vi "CC Install Simulation Config File.vi"() -> (2 "Hardware Config out":T1, 3 "new path":path)   [LabVIEW 2024]
uses:
  typedefs/CC cluster Hardware Config.ctl
  typedefs/CC cluster Device Index.ctl
panel:
  in  "OK Button":bool
  in  "Select Install Type":enum16{"Simulation", "Full Standard Hardware"}(ring)
  # "RIMAS Camera Control"
  # "No configuration file found. Select configuration from list below. Simulation mode will simulate all subsystem hardware. Full Standard Hardware attempts to communicate with all subsystems.\n\nHardware selections can be changed at anytime using the Settings-->Select Hardware menu option."
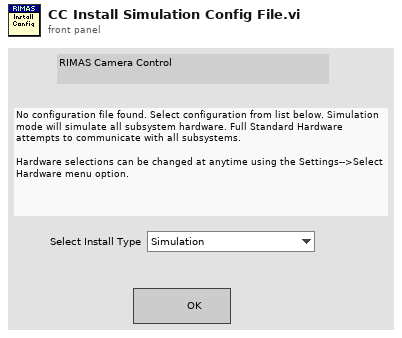
[diagram p1: front panel]
types:
  T1 = typedef "CC cluster Hardware Config.ctl" = cluster{"Installed Hardware":T2[]}
  T2 = typedef "CC cluster Device Index.ctl" = cluster{"Device Type Name":string, "Curr Device Name":string, "All Instances":string[]}
  T3 = enum32{"Invalid", "Standard", "Closed", "Hidden", "Minimized", "Maximized"}
diagram:
  w1 = "{\n  \"Arduino Focus Settings\":{\n    \"Homed\":[true,true],\n    \"Homing Parameters\":{\n      \"ACC/DECEL STEPS/SEC^2\":1000,\n      \"Direction\":false,\n      \"EN/DIS?\":true,\n      \"NUMBER OF  STEPS\":13000,\n      \"SPEED STEPS/SEC\":1000\n    },\n    \"Port\":\"ArduinoFocus\",\n    \"Positions\":[300,200]\n  },\n  \"Cryo Alarms\":{\n    \"Enabled\":false,\n    \"Reject Shutdown Temp\":40,\n    \"Reject Temp Warning\":20,\n    \"Temperature Error Max\":4\n  },\n  \"CryoCooler Settings\":{\n    \"Cryo Addr\":[\"Cooler1\",\"Cooler2\",\"Cooler3\"]\n  },\n  \"Detector Config PRIME\":{\"Detector\":0,\"Offsets\":[[0,0,0,0,0,0,0,0,0,0,0,0,0,0,0,0,0,0,0,0,0,0,0,0,0,0,0,0,0,0,0,0]],\"Detector Computer\":{\"Machine\":\"127.0.0.1\",\"Password\":\"R!MAS1grb\",\"FITS File Path\":\"/local/data/fermi-grb1/home/rimas/dev/h2rg/fitdat\",\"Port\":20750,\"Header Path\":\"/local/data/fermi-grb1/home/rimas/dev/h2rg/header\",\"Name\":\"PRIME\"},\"FITS hdr template0\":\"C:\\\\Users\\\\gsfcprime\\\\Documents\\\\LabVIEW Data\\\\FITS Templates\\\\header0.dat\",\"FITS hdr template1\":\"C:\\\\Users\\\\gsfcprime\\\\Documents\\\\LabVIEW Data\\\\FITS Templates\\\\header1.dat\",\"FITS Data File Path\":\"C:\\\\Users\\\\gsfcprime\\\\Documents\\\\LabVIEW Data\\\\PRIME FITS Images\",\"FITS Detector Settings\":{\"Exp Time Short\":1,\"# of Frames\":1,\"Exp Time Long\":2,\"# of Groups\":1,\"Object Name\":\"Auto\",\"Object\":\"\",\"Obs Type\":\"\",\"Image Type\":\"\",\"Observer\":\"\",\"Observer Affiliation\":\"\"},\"Sim Folder\":\"C:\\\\Users\\\\gsfcprime\\\\Documents\\\\LabVIEW Data\\\\PRIME Simulation FITS Images\",\"Integration Mode\":\"CDS\",\"Integration Time\":300,\"Frame Int Time\":3},\n  \"Detector Config RIMAS\":{\n    \"Detector Computer\":{\n      \"FITS File Path\":\"/local/data/fermi-grb1/home/rimas/dev/h2rg/fitdat\",\n      \"Header Path\":\"/local/data/fermi-grb1/home/rimas/dev/h2rg/header\",\n      \"Machine\":\"192.168.121.11\",\n      \"Name\":\"RIMAS\",\n      \"Password\":\"R!MAS1grb\",\n      \"Port\":44444\n    },\n    \"Detector\":0,\n    \"FITS Data File Path\":\"C:\\\\Users\\\\gsfcprime\\\\Documents\\\\LabVIEW Data\\\\PRIME FITS Images\",\n    \"FITS Detector Settings\":{\n      \"# of Frames\":1,\n      \"# of Groups\":1,\n      \"Exp Time Long\":2,\n      \"Exp Time Short\":1,\n      \"Image Type\":\"\",\n      \"Object Name\":\"\",\n      \"Object\":\"\",\n      \"Obs Type\":\"\",\n      \"Observer Affiliation\":\"\",\n      \"Observer\":\"\"\n    },\n    \"FITS hdr template0\":\"C:\\\\Users\\\\gsfcprime\\\\Documents\\\\LabVIEW Data\\\\FITS Templates\\\\header0.dat\",\n    \"FITS hdr template1\":\"C:\\\\Users\\\\gsfcprime\\\\Documents\\\\LabVIEW Data\\\\FITS Templates\\\\header1.dat\",\n    \"Frame Int Time\":0,\n    \"Integration Mode\":\"SSR\",\n    \"Integration Time\":0,\n    \"Offsets\":[\n      [\n        0,\n        0,\n        0,\n        0,\n        0,\n        0,\n        0,\n        0,\n        0,\n        0,\n        0,\n        0,\n        0,\n        0,\n        0,\n        0,\n        0,\n        0,\n        0,\n        0,\n        0,\n        0,\n        0,\n        0,\n        0,\n        0,\n        0,\n        0,\n        0,\n        0,\n        0,\n        0\n      ]\n    ],\n    \"Sim Folder\":\"C:\\\\Users\\\\gsfcprime\\\\Documents\\\\LabVIEW Data\\\\PRIME Simulation FITS Images\"\n  },\n  \"Detector Config Simulation\":{\n    \"Detector Computer\":{\n      \"FITS File Path\":\"/local/data/fermi-grb1/home/rimas/dev/h2rg/fitdat\",\n      \"Header Path\":\"/local/data/fermi-grb1/home/rimas/dev/h2rg/header\",\n      \"Machine\":\"\",\n      \"Name\":\"Simulation\",\n      \"Password\":\"R!MAS1grb\",\n      \"Port\":44444\n    },\n    \"Detector\":0,\n    \"FITS Data File Path\":\"C:\\\\Users\\\\gsfcprime\\\\Documents\\\\LabVIEW Data\\\\PRIME FITS Images\",\n    \"FITS Detector Settings\":{\n      \"# of Frames\":1,\n      \"# of Groups\":1,\n      \"Exp Time Long\":2,\n      \"Exp Time Short\":1,\n      \"Image Type\":\"\",\n      \"Object Name\":\"\",\n      \"Object\":\"\",\n      \"Obs Type\":\"\",\n      \"Observer Affiliation\":\"\",\n      \"Observer\":\"\"\n    },\n    \"FITS hdr template0\":\"C:\\\\Users\\\\gsfcprime\\\\Documents\\\\LabVIEW Data\\\\FITS Templates\\\\header0.dat\",\n    \"FITS hdr template1\":\"C:\\\\Users\\\\gsfcprime\\\\Documents\\\\LabVIEW Data\\\\FITS Templates\\\\header1.dat\",\n    \"Frame Int Time\":10,\n    \"Integration Mode\":\"SSR\",\n    \"Integration Time\":0,\n    \"Offsets\":[\n      [\n        0,\n        0,\n        0,\n        0,\n        0,\n        0,\n        0,\n        0,\n        0,\n        0,\n        0,\n        0,\n        0,\n        0,\n        0,\n        0,\n        0,\n        0,\n        0,\n        0,\n        0,\n        0,\n        0,\n        0,\n        0,\n        0,\n        0,\n        0,\n        0,\n        0,\n        0,\n        0\n      ]\n    ],\n    \"Sim Folder\":\"C:\\\\Users\\\\gsfcprime\\\\Documents\\\\LabVIEW Data\\\\PRIME Simulation FITS Images\"\n  },\n  \"Filter Wheel Settings RIMAS\":{\n    \"Addr\":\"ArduinoFilter\",\n    \"Default Speed\":200,\n    \"Filters\":[\n      {\n        \"Names\":[\"Grism\",\"Open\",\"Vph30\",\"Vph300\",\"Y\",\"J\"],\n        \"Relative Position\":[0,10000,17000,25000,33000,40000],\n        \"Size\":50000,\n        \"Wheel Name\":\"FW YJ\"\n      },\n      {\n        \"Names\":[\"Grism\",\"Open\",\"Vph30\",\"Vph300\",\"H\",\"K\"],\n        \"Relative Position\":[0,10000,17000,25000,33000,40000],\n        \"Size\":50000,\n        \"Wheel Name\":\"FW HK\"\n      },\n      {\n        \"Names\":[\n          \"K\",\n          \"Open\",\n          \"blank\",\n          \"Br-g\",\n          \"H2\",\n          \"2180\",\n          \"2190\"\n        ],\n        \"Relative Position\":[0,5560,11809,17908,23466,29016,34579],\n        \"Size\":40141,\n        \"Wheel Name\":\"Aux\"\n      },\n      {\n        \"Names\":[\n          \"blank\",\n          \"long\",\n          \"250 um\",\n          \"130 um\",\n          \"80 um\",\n          \"open\"\n        ],\n        \"Relative Position\":[0,5667,12889,20111,27333,34222],\n        \"Size\":40000,\n        \"Wheel Name\":\"Slit\"\n      }\n    ],\n    \"Homing\":[\n      {\n        \"Accel\":267,\n        \"Direction\":true,\n        \"Error Cnts\":300,\n        \"Homing Delta\":3000,\n        \"Speed\":400\n      },\n      {\n        \"Accel\":160,\n        \"Direction\":true,\n        \"Error Cnts\":1000,\n        \"Homing Delta\":4000,\n        \"Speed\":400\n      },\n      {\n        \"Accel\":600,\n        \"Direction\":true,\n        \"Error Cnts\":200,\n        \"Homing Delta\":-680,\n        \"Speed\":400\n      },\n      {\n        \"Accel\":800,\n        \"Direction\":true,\n        \"Error Cnts\":300,\n        \"Homing Delta\":-1560,\n        \"Speed\":400\n      }\n    ],\n    \"Invalid Combinations\":[[]],\n    \"Name\":\"RIMAS\",\n    \"Num Wheels\":4,\n    \"Simulate\":false\n  },\n  \"Filter Wheel Settings Simulation\":{\n    \"Addr\":\"COM15\",\n    \"Default Speed\":200,\n    \"Filters\":[\n      {\n        \"Names\":[\"Grism\",\"blocked\",\"open\",\"VPH\",\"J\",\"Y\"],\n        \"Relative Position\":[10000,7000,8000,8000,7000,10000],\n        \"Wheel Name\":\"FW YJ\"\n      },\n      {\n        \"Names\":[\"Grism\",\"blocked\",\"open\",\"VPH\",\"H\",\"K\"],\n        \"Relative Position\":[10000,7000,8000,8000,7000,10000],\n        \"Wheel Name\":\"FW HK\"\n      },\n      {\n        \"Names\":[\n          \"135\",\n          \"blocked\",\n          \"80\",\n          \"open 1\",\n          \"250\",\n          \"open\"\n        ],\n        \"Relative Position\":[6000,6000,7000,7000,7000,7000],\n        \"Wheel Name\":\"Slit wheel\"\n      },\n      {\n        \"Names\":[\"A\",\"B\",\"C\",\"D\",\"E\",\"F\",\"G\",\"H\"],\n        \"Relative Position\":[5000,5000,5000,5000,5000,5000,5000,5000],\n        \"Wheel Name\":\"FW aux\"\n      }\n    ],\n    \"Homing Parameters\":{\n      \"Accel\":400,\n      \"Direction (F: CW)\":true,\n      \"Error Cnts\":100,\n      \"Homing Deltas\":[3000,3000,-680,-1560],\n      \"Speed\":150\n    },\n    \"Invalid Combinations\":[[]],\n    \"Name\":\"Simulation\",\n    \"Num Wheels\":4,\n    \"Simulate\":true\n  },\n  \"Focus Settings Arduino\":{\n    \"Last Positions\":[0,0],\n    \"Motion Settings\":{\n      \"Steps Per Sec 2\":100,\n      \"Steps Per Sec\":100\n    },\n    \"Type\":\"Arduino\"\n  },\n  \"Focus Settings Default\":{\"Type\":\"Arduino\",\"Motion Settings\":{\"Steps Per Sec\":100,\"Steps Per Sec 2\":100},\"Last Positions\":[300,200]},\n  \"Hardware Settings\":{\n    \"Installed Hardware\":[\n      {\n        \"All Instances\":[\"Simulation\",\"RIMAS\"],\n        \"Curr Device Name\":\"RIMAS\",\n        \"Device Type Name\":\"filter wheel\"\n      },\n      {\n        \"All Instances\":[\"Simulation\",\"Lakeshore 325\"],\n        \"Curr Device Name\":\"Lakeshore 325\",\n        \"Device Type Name\":\"temp control 1\"\n      },\n      {\n        \"All Instances\":[\"simulation\",\"Lakeshore 331\"],\n        \"Curr Device Name\":\"Lakeshore 331\",\n        \"Device Type Name\":\"temp control 2\"\n      },\n      {\n        \"All Instances\":[\"Simulation\",\"Lowell\",\"PRIME\"],\n        \"Curr Device Name\":\"Simulation\",\n        \"Device Type Name\":\"telescope\"\n      },\n      {\n        \"All Instances\":[\"Simulation\",\"Lakeshore 218\"],\n        \"Curr Device Name\":\"Lakeshore 218\",\n        \"Device Type Name\":\"temp control 3\"\n      },\n      {\n        \"All Instances\":[\"Simulation\",\"Arduino\",\"New Focus\"],\n        \"Curr Device Name\":\"Arduino\",\n        \"Device Type Name\":\"focus\"\n      },\n      {\n        \"All Instances\":[\"Simulation\",\"Lesker\"],\n        \"Curr Device Name\":\"Lesker\",\n        \"Device Type Name\":\"pressure monitor\"\n      },\n      {\n        \"All Instances\":[\"Simulation\",\"RIMAS\"],\n        \"Curr Device Name\":\"RIMAS\",\n        \"Device Type Name\":\"cryocooler\"\n      },\n      {\n        \"All Instances\":[\"Simulation\",\"RIMAS\",\"PRIME\"],\n        \"Curr Device Name\":\"PRIME\",\n        \"Device Type Name\":\"detector\"\n      }\n    ]\n  },\n  \"Homing Parameters\":{\n    \"Accel\":400,\n    \"Direction (F: CW)\":true,\n    \"Error Cnts\":300,\n    \"Homing Deltas\":[3000,3250,-680,-1560],\n    \"Speed\":200\n  },\n  \"Homing\":[\n    {\n      \"Accel\":267,\n      \"Direction\":true,\n      \"Error Cnts\":300,\n      \"Homing Delta\":3000,\n      \"Speed\":400\n    },\n    {\n      \"Accel\":160,\n      \"Direction\":true,\n      \"Error Cnts\":1000,\n      \"Homing Delta\":4000,\n      \"Speed\":400\n    },\n    {\n      \"Accel\":600,\n      \"Direction\":true,\n      \"Error Cnts\":300,\n      \"Homing Delta\":-680,\n      \"Speed\":400\n    },\n    {\n      \"Accel\":800,\n      \"Direction\":true,\n      \"Error Cnts\":300,\n      \"Homing Delta\":-1560,\n      \"Speed\":400\n    }\n  ],\n  \"LDT Telescope Settings\":{\n    \"host\":\"tanagra.lowell.edu\",\n    \"port\":\"61616\"\n  },\n  \"Lakeshore 331 Parameters\":{\n    \"Control Parameters\":{\"D\":0,\"I\":17,\"P\":80},\n    \"Default Range\":1,\n    \"Heater Range\":1,\n    \"Manual Power (%)\":20,\n    \"Mode\":0,\n    \"Setpoint\":97\n  },\n  \"Lakeshore 331\":{\n    \"Addr\":\"Lakeshore-331\",\n    \"Ch Prefix\":\"LS331\",\n    \"Ch Select\":[]\n  },\n  \"Lakeshore331\":{\n    \"Addr\":\"GPIB0::12::INSTR\",\n    \"Ch Prefix\":\"\",\n    \"Ch Select\":[]\n  },\n  \"Orion Parameters rimas pdu1\":{\n    \"Password\":\"infrared\",\n    \"URL\":\"192.168.121.218\",\n    \"Username\":\"rimas\"\n  },\n  \"Orion Parameters rimas pdu2\":{\n    \"Password\":\"infrared\",\n    \"URL\":\"192.168.121.216\",\n    \"Username\":\"rimas\"\n  },\n  \"Orion Parameters test program\":{\n    \"Password\":\"infrared\",\n    \"URL\":\"192.168.121.218\",\n    \"Username\":\"rimas\"\n  },\n  \"Orion Parameters\":{\n    \"Password\":\"infrared\",\n    \"URL\":\"192.168.121.218\",\n    \"Username\":\"rimas\"\n  },\n  \"PRIME Detector Settings\":{\n    \"Python Server\":\"C:\\\\PycharmProjects\\\\asdetector\"\n  },\n  \"Pressur Monitor Settings\":{\n    \"Enabled?\":[true,false],\n    \"Filaments\":[],\n    \"Lesker Addrs\":[\"Lesker\",\"COM20\"],\n    \"Pressure Alarm Level\":0.001\n  },\n  \"System Settings\":{\n    \"HK Table Name\":\"\",\n    \"Images Folder\":\"E:\\\\asdetector-data\\\\output\\\\raw\\\\20240223\",\n    \"Obs File\":\"C:\\\\Users\\\\gsfcprime\\\\Documents\\\\LabVIEW Data\\\\Jan12_2024.csv\"\n  },\n  \"WebRelay10 Settings\":{\n    \"Address\":\"192.168.121.216\",\n    \"Names\":[],\n    \"Port\":80\n  }\n}"  # Master
  w2 = "{\n  \"Arduino Focus Settings\":{\n    \"Homed\":[true,true],\n    \"Homing Parameters\":{\n      \"ACC/DECEL STEPS/SEC^2\":1000,\n      \"Direction\":false,\n      \"EN/DIS?\":true,\n      \"NUMBER OF  STEPS\":13000,\n      \"SPEED STEPS/SEC\":1000\n    },\n    \"Port\":\"ArduinoFocus\",\n    \"Positions\":[300,200]\n  },\n  \"Cryo Alarms\":{\n    \"Enabled\":false,\n    \"Reject Shutdown Temp\":40,\n    \"Reject Temp Warning\":20,\n    \"Temperature Error Max\":4\n  },\n  \"CryoCooler Settings\":{\n    \"Cryo Addr\":[\"Cooler1\",\"Cooler2\",\"Cooler3\"]\n  },\n  \"Detector Config PRIME\":{\"Detector\":0,\"Offsets\":[[0,0,0,0,0,0,0,0,0,0,0,0,0,0,0,0,0,0,0,0,0,0,0,0,0,0,0,0,0,0,0,0]],\"Detector Computer\":{\"Machine\":\"127.0.0.1\",\"Password\":\"R!MAS1grb\",\"FITS File Path\":\"/local/data/fermi-grb1/home/rimas/dev/h2rg/fitdat\",\"Port\":20750,\"Header Path\":\"/local/data/fermi-grb1/home/rimas/dev/h2rg/header\",\"Name\":\"PRIME\"},\"FITS hdr template0\":\"C:\\\\Users\\\\gsfcprime\\\\Documents\\\\LabVIEW Data\\\\FITS Templates\\\\header0.dat\",\"FITS hdr template1\":\"C:\\\\Users\\\\gsfcprime\\\\Documents\\\\LabVIEW Data\\\\FITS Templates\\\\header1.dat\",\"FITS Data File Path\":\"C:\\\\Users\\\\gsfcprime\\\\Documents\\\\LabVIEW Data\\\\PRIME FITS Images\",\"FITS Detector Settings\":{\"Exp Time Short\":1,\"# of Frames\":1,\"Exp Time Long\":2,\"# of Groups\":1,\"Object Name\":\"Auto\",\"Object\":\"\",\"Obs Type\":\"\",\"Image Type\":\"\",\"Observer\":\"\",\"Observer Affiliation\":\"\"},\"Sim Folder\":\"C:\\\\Users\\\\gsfcprime\\\\Documents\\\\LabVIEW Data\\\\PRIME Simulation FITS Images\",\"Integration Mode\":\"CDS\",\"Integration Time\":9,\"Frame Int Time\":3},\n  \"Detector Config RIMAS\":{\n    \"Detector Computer\":{\n      \"FITS File Path\":\"/local/data/fermi-grb1/home/rimas/dev/h2rg/fitdat\",\n      \"Header Path\":\"/local/data/fermi-grb1/home/rimas/dev/h2rg/header\",\n      \"Machine\":\"192.168.121.11\",\n      \"Name\":\"RIMAS\",\n      \"Password\":\"R!MAS1grb\",\n      \"Port\":44444\n    },\n    \"Detector\":0,\n    \"FITS Data File Path\":\"C:\\\\Users\\\\gsfcprime\\\\Documents\\\\LabVIEW Data\\\\PRIME FITS Images\",\n    \"FITS Detector Settings\":{\n      \"# of Frames\":1,\n      \"# of Groups\":1,\n      \"Exp Time Long\":2,\n      \"Exp Time Short\":1,\n      \"Image Type\":\"\",\n      \"Object Name\":\"\",\n      \"Object\":\"\",\n      \"Obs Type\":\"\",\n      \"Observer Affiliation\":\"\",\n      \"Observer\":\"\"\n    },\n    \"FITS hdr template0\":\"C:\\\\Users\\\\gsfcprime\\\\Documents\\\\LabVIEW Data\\\\FITS Templates\\\\header0.dat\",\n    \"FITS hdr template1\":\"C:\\\\Users\\\\gsfcprime\\\\Documents\\\\LabVIEW Data\\\\FITS Templates\\\\header1.dat\",\n    \"Frame Int Time\":0,\n    \"Integration Mode\":\"SSR\",\n    \"Integration Time\":0,\n    \"Offsets\":[\n      [\n        0,\n        0,\n        0,\n        0,\n        0,\n        0,\n        0,\n        0,\n        0,\n        0,\n        0,\n        0,\n        0,\n        0,\n        0,\n        0,\n        0,\n        0,\n        0,\n        0,\n        0,\n        0,\n        0,\n        0,\n        0,\n        0,\n        0,\n        0,\n        0,\n        0,\n        0,\n        0\n      ]\n    ],\n    \"Sim Folder\":\"C:\\\\Users\\\\gsfcprime\\\\Documents\\\\LabVIEW Data\\\\PRIME Simulation FITS Images\"\n  },\n  \"Detector Config Simulation\":{\n    \"Detector Computer\":{\n      \"FITS File Path\":\"/local/data/fermi-grb1/home/rimas/dev/h2rg/fitdat\",\n      \"Header Path\":\"/local/data/fermi-grb1/home/rimas/dev/h2rg/header\",\n      \"Machine\":\"\",\n      \"Name\":\"Simulation\",\n      \"Password\":\"R!MAS1grb\",\n      \"Port\":44444\n    },\n    \"Detector\":0,\n    \"FITS Data File Path\":\"C:\\\\Users\\\\gsfcprime\\\\Documents\\\\LabVIEW Data\\\\PRIME FITS Images\",\n    \"FITS Detector Settings\":{\n      \"# of Frames\":1,\n      \"# of Groups\":1,\n      \"Exp Time Long\":2,\n      \"Exp Time Short\":1,\n      \"Image Type\":\"\",\n      \"Object Name\":\"\",\n      \"Object\":\"\",\n      \"Obs Type\":\"\",\n      \"Observer Affiliation\":\"\",\n      \"Observer\":\"\"\n    },\n    \"FITS hdr template0\":\"C:\\\\Users\\\\gsfcprime\\\\Documents\\\\LabVIEW Data\\\\FITS Templates\\\\header0.dat\",\n    \"FITS hdr template1\":\"C:\\\\Users\\\\gsfcprime\\\\Documents\\\\LabVIEW Data\\\\FITS Templates\\\\header1.dat\",\n    \"Frame Int Time\":10,\n    \"Integration Mode\":\"SSR\",\n    \"Integration Time\":0,\n    \"Offsets\":[\n      [\n        0,\n        0,\n        0,\n        0,\n        0,\n        0,\n        0,\n        0,\n        0,\n        0,\n        0,\n        0,\n        0,\n        0,\n        0,\n        0,\n        0,\n        0,\n        0,\n        0,\n        0,\n        0,\n        0,\n        0,\n        0,\n        0,\n        0,\n        0,\n        0,\n        0,\n        0,\n        0\n      ]\n    ],\n    \"Sim Folder\":\"C:\\\\Users\\\\gsfcprime\\\\Documents\\\\LabVIEW Data\\\\PRIME Simulation FITS Images\"\n  },\n  \"Filter Wheel Settings RIMAS\":{\n    \"Addr\":\"COM15\",\n    \"Default Speed\":200,\n    \"Filters\":[\n      {\n        \"Names\":[\"Grism\",\"Open\",\"Vph30\",\"Vph300\",\"Y\",\"J\"],\n        \"Relative Position\":[0,10000,17000,25000,33000,40000],\n        \"Size\":50000,\n        \"Wheel Name\":\"FW YJ\"\n      },\n      {\n        \"Names\":[\"Grism\",\"Open\",\"Vph30\",\"Vph300\",\"H\",\"K\"],\n        \"Relative Position\":[0,10000,17000,25000,33000,40000],\n        \"Size\":50000,\n        \"Wheel Name\":\"FW HK\"\n      },\n      {\n        \"Names\":[\n          \"K\",\n          \"Open\",\n          \"blank\",\n          \"Br-g\",\n          \"H2\",\n          \"2180\",\n          \"2190\"\n        ],\n        \"Relative Position\":[0,5560,11809,17908,23466,29016,34579],\n        \"Size\":40141,\n        \"Wheel Name\":\"Aux\"\n      },\n      {\n        \"Names\":[\n          \"blank\",\n          \"long\",\n          \"250 um\",\n          \"130 um\",\n          \"80 um\",\n          \"open\"\n        ],\n        \"Relative Position\":[0,5667,12889,20111,27333,34222],\n        \"Size\":40000,\n        \"Wheel Name\":\"Slit\"\n      }\n    ],\n    \"Homing\":[\n      {\n        \"Accel\":267,\n        \"Direction\":true,\n        \"Error Cnts\":300,\n        \"Homing Delta\":3000,\n        \"Speed\":400\n      },\n      {\n        \"Accel\":160,\n        \"Direction\":true,\n        \"Error Cnts\":300,\n        \"Homing Delta\":3250,\n        \"Speed\":400\n      },\n      {\n        \"Accel\":600,\n        \"Direction\":true,\n        \"Error Cnts\":300,\n        \"Homing Delta\":-680,\n        \"Speed\":400\n      },\n      {\n        \"Accel\":800,\n        \"Direction\":true,\n        \"Error Cnts\":300,\n        \"Homing Delta\":-1560,\n        \"Speed\":400\n      }\n    ],\n    \"Invalid Combinations\":[[]],\n    \"Name\":\"RIMAS\",\n    \"Num Wheels\":4,\n    \"Simulate\":false\n  },\n  \"Filter Wheel Settings Simulation\":{\n    \"Addr\":\"COM15\",\n    \"Default Speed\":200,\n    \"Filters\":[\n      {\n        \"Names\":[\"Grism\",\"blocked\",\"open\",\"VPH\",\"J\",\"Y\"],\n        \"Relative Position\":[10000,7000,8000,8000,7000,10000],\n        \"Wheel Name\":\"FW YJ\"\n      },\n      {\n        \"Names\":[\"Grism\",\"blocked\",\"open\",\"VPH\",\"H\",\"K\"],\n        \"Relative Position\":[10000,7000,8000,8000,7000,10000],\n        \"Wheel Name\":\"FW HK\"\n      },\n      {\n        \"Names\":[\n          \"135\",\n          \"blocked\",\n          \"80\",\n          \"open 1\",\n          \"250\",\n          \"open\"\n        ],\n        \"Relative Position\":[6000,6000,7000,7000,7000,7000],\n        \"Wheel Name\":\"Slit wheel\"\n      },\n      {\n        \"Names\":[\"A\",\"B\",\"C\",\"D\",\"E\",\"F\",\"G\",\"H\"],\n        \"Relative Position\":[5000,5000,5000,5000,5000,5000,5000,5000],\n        \"Wheel Name\":\"FW aux\"\n      }\n    ],\n    \"Homing Parameters\":{\n      \"Accel\":400,\n      \"Direction (F: CW)\":true,\n      \"Error Cnts\":100,\n      \"Homing Deltas\":[3000,3000,-680,-1560],\n      \"Speed\":150\n    },\n    \"Invalid Combinations\":[[]],\n    \"Name\":\"Simulation\",\n    \"Num Wheels\":4,\n    \"Simulate\":true\n  },\n  \"Focus Settings Arduino\":{\n    \"Last Positions\":[0,0],\n    \"Motion Settings\":{\n      \"Steps Per Sec 2\":100,\n      \"Steps Per Sec\":100\n    },\n    \"Type\":\"Arduino\"\n  },\n  \"Focus Settings Default\":{\n    \"Last Positions\":[300,200],\n    \"Motion Settings\":{\n      \"Steps Per Sec 2\":100,\n      \"Steps Per Sec\":100\n    },\n    \"Type\":\"Arduino\"\n  },\n  \"Hardware Settings\":{\n    \"Installed Hardware\":[\n      {\n        \"All Instances\":[\"Simulation\",\"RIMAS\"],\n        \"Curr Device Name\":\"Simulation\",\n        \"Device Type Name\":\"filter wheel\"\n      },\n      {\n        \"All Instances\":[\"Simulation\",\"Lakeshore 325\"],\n        \"Curr Device Name\":\"Simulation\",\n        \"Device Type Name\":\"temp control 1\"\n      },\n      {\n        \"All Instances\":[\"simulation\",\"Lakeshore 331\"],\n        \"Curr Device Name\":\"simulation\",\n        \"Device Type Name\":\"temp control 2\"\n      },\n      {\n        \"All Instances\":[\"Simulation\",\"Lowell\",\"PRIME\"],\n        \"Curr Device Name\":\"Simulation\",\n        \"Device Type Name\":\"telescope\"\n      },\n      {\n        \"All Instances\":[\"Simulation\",\"Lakeshore 218\"],\n        \"Curr Device Name\":\"Simulation\",\n        \"Device Type Name\":\"temp control 3\"\n      },\n      {\n        \"All Instances\":[\"Simulation\",\"Arduino\",\"New Focus\"],\n        \"Curr Device Name\":\"Simulation\",\n        \"Device Type Name\":\"focus\"\n      },\n      {\n        \"All Instances\":[\"Simulation\",\"Lesker\"],\n        \"Curr Device Name\":\"Simulation\",\n        \"Device Type Name\":\"pressure monitor\"\n      },\n      {\n        \"All Instances\":[\"Simulation\",\"RIMAS\"],\n        \"Curr Device Name\":\"Simulation\",\n        \"Device Type Name\":\"cryocooler\"\n      },\n      {\n        \"All Instances\":[\"Simulation\",\"RIMAS\",\"PRIME\"],\n        \"Curr Device Name\":\"Simulation\",\n        \"Device Type Name\":\"detector\"\n      }\n    ]\n  },\n  \"Homing Parameters\":{\n    \"Accel\":400,\n    \"Direction (F: CW)\":true,\n    \"Error Cnts\":300,\n    \"Homing Deltas\":[3000,3250,-680,-1560],\n    \"Speed\":200\n  },\n  \"Homing\":[\n    {\n      \"Accel\":400,\n      \"Direction\":true,\n      \"Error Cnts\":300,\n      \"Homing Delta\":3000,\n      \"Speed\":400\n    },\n    {\n      \"Accel\":400,\n      \"Direction\":true,\n      \"Error Cnts\":300,\n      \"Homing Delta\":3250,\n      \"Speed\":400\n    },\n    {\n      \"Accel\":400,\n      \"Direction\":true,\n      \"Error Cnts\":300,\n      \"Homing Delta\":-680,\n      \"Speed\":400\n    },\n    {\n      \"Accel\":400,\n      \"Direction\":true,\n      \"Error Cnts\":300,\n      \"Homing Delta\":-1560,\n      \"Speed\":400\n    }\n  ],\n  \"LDT Telescope Settings\":{\n    \"host\":\"tanagra.lowell.edu\",\n    \"port\":\"61616\"\n  },\n  \"Lakeshore 331 Parameters\":{\n    \"Control Parameters\":{\"D\":0,\"I\":17,\"P\":80},\n    \"Default Range\":1,\n    \"Heater Range\":1,\n    \"Manual Power (%)\":20,\n    \"Mode\":0,\n    \"Setpoint\":97\n  },\n  \"Lakeshore 331\":{\n    \"Addr\":\"Lakeshore-331\",\n    \"Ch Prefix\":\"LS331\",\n    \"Ch Select\":[]\n  },\n  \"Lakeshore331\":{\n    \"Addr\":\"GPIB0::12::INSTR\",\n    \"Ch Prefix\":\"\",\n    \"Ch Select\":[]\n  },\n  \"Orion Parameters rimas pdu1\":{\n    \"Password\":\"infrared\",\n    \"URL\":\"192.168.121.218\",\n    \"Username\":\"rimas\"\n  },\n  \"Orion Parameters rimas pdu2\":{\n    \"Password\":\"infrared\",\n    \"URL\":\"192.168.121.216\",\n    \"Username\":\"rimas\"\n  },\n  \"Orion Parameters test program\":{\n    \"Password\":\"infrared\",\n    \"URL\":\"192.168.121.218\",\n    \"Username\":\"rimas\"\n  },\n  \"Orion Parameters\":{\n    \"Password\":\"infrared\",\n    \"URL\":\"192.168.121.218\",\n    \"Username\":\"rimas\"\n  },\n  \"PRIME Detector Settings\":{\n    \"Python Server\":\"C:\\\\PycharmProjects\\\\asdetector\"\n  },\n  \"Pressur Monitor Settings\":{\n    \"Enabled?\":[true,false],\n    \"Filaments\":[],\n    \"Lesker Addrs\":[\"Lesker\",\"\"],\n    \"Pressure Alarm Level\":10\n  },\n  \"System Settings\":{\n    \"HK Table Name\":\"\",\n    \"Images Folder\":\"E:\\\\asdetector-data\\\\output\\\\raw\\\\20240112\",\n    \"Obs File\":\"\"\n  },\n  \"WebRelay10 Settings\":{\n    \"Address\":\"192.168.121.216\",\n    \"Names\":[],\n    \"Port\":80\n  }\n}"  # Simulation
  n1 = call "CC Rd Wr Hardware Configuration.vi"() -> ("New File?"=w7:bool, "File"=w5:path, "Hardware Config out"=w6:T1)  [unwired: 8 in, 1 out]
  n2 = case shown="True" w7 {
    tunnel: w6 -> [w8 _]
    tunnel: w5 -> [w9 w11]
    tunnel: w2 -> [_ w19]
    tunnel: w1 -> [_ w18]
    tunnel: [w9 w11] -> w4
    tunnel: [w8 w16] -> w3
    frame False {
    }
    frame True {
      n3 = invoke class="VI" method="FP.Open"("Activate"=TRUE ("Activate?")) -> (reference out=w15:refnum<vi>, error out=w10:errorcluster)  [unwired: 4 in, 3 out]
      n4 = while {
        tunnel: ["Select Install Type"] -> w22
        tunnel: w10 -> [_]
        stop <- "OK Button" stop-if-true
        n5 = Wait Until Next ms Multiple(millisecond multiple=u32 20) -> ()  [unwired: 1 out]
      }
      n6 = Equal?(x=w22, y=enum16{"Simulation", "Full Standard Hardware"}."Simulation") -> (x = y?=w20:bool)
      n7 = Select(t=w19, s=w20, f=w18) -> (s? t:f=w13:string)
      n8 = Write to Text File(file (use dialog)=w11, text=w13) -> (error out=w12:errorcluster)  [unwired: 2 in, 2 out]
      n9 = property class="VI"(reference=w15, error in=w12, "FP.State"=T3."Closed" ("Front Panel Window:State")) -> ()  [unwired: 2 out]
      n10 = call "CC Rd Wr Hardware Configuration.vi"("error in (no error)"=w12) -> ("Hardware Config out"=w16:T1)  [unwired: 7 in, 3 out]
    }
  }
  "new path" <- w4
  "Hardware Config out" <- w3
